vi "Gen VIs.vi"(8 "error in (no error)":errorcluster, 11 "Progress":refnum<vi>) -> (0 "error out":errorcluster, 3 "Progress (out)":refnum<vi>)   [LabVIEW 2020, in "WebServiceImporter.lvlib" / "VI Generator.lvlib"]
uses:
  <vilib>/Platform/WebService/VI Generator/VI Generator.lvlib
  <vilib>/Platform/WebService/Global/Const Strings.vi
  <vilib>/Platform/WebService/Main Panel/Pages/Progress/Progress.lvlib
  <vilib>/Platform/WebService/WebServiceImporter.lvlib
  <vilib>/Platform/WebService/ProxyDll Generator/ProxyDll Generator.lvlib
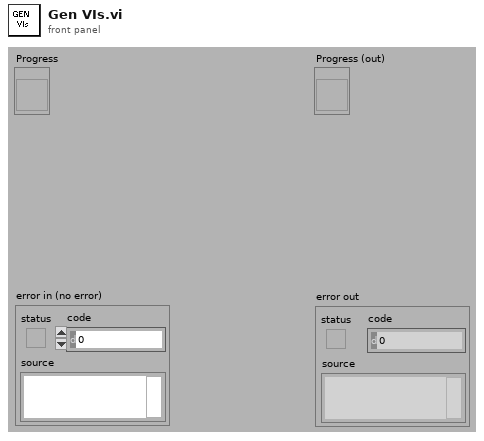
[diagram p1: front panel]
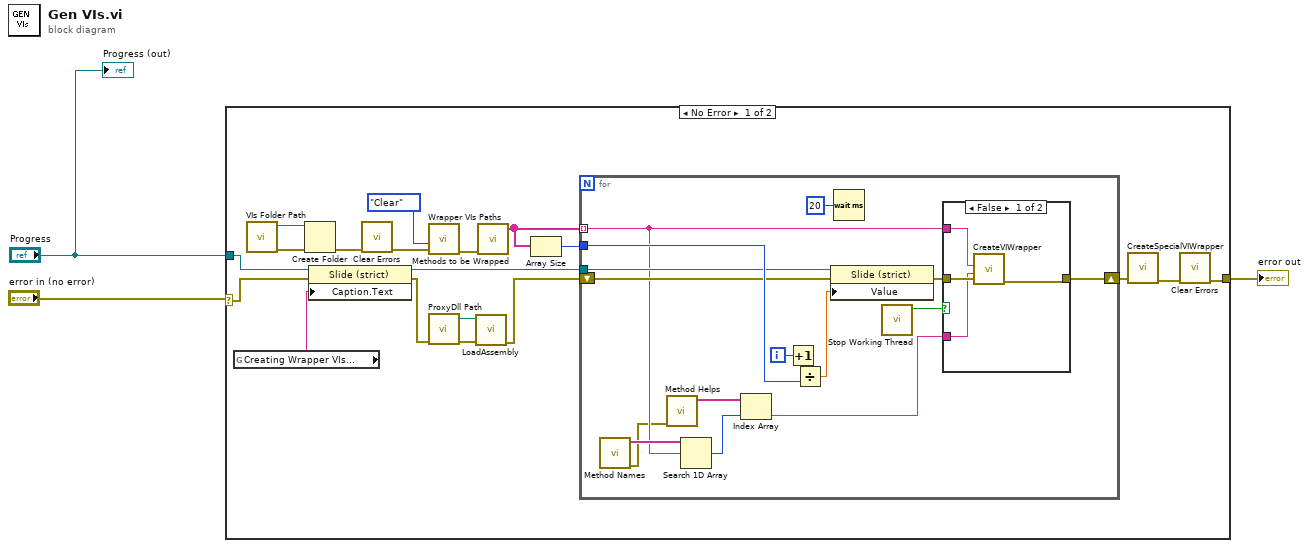
[diagram p0: block diagram]
diagram:
  n1 = case shown="No Error" "error in (no error)" {
    selector: "error in (no error)" -> [w18 w44]
    tunnel: "Progress" -> [w19 _]
    tunnel: [w13 w44] -> w2
    frame No Error {
      n2 = global read "Const Strings.vi" "Creating Wrapper VIs..."() -> (w10:string)
      n3 = call <vilib>:"VIs Folder Path.vi"() -> ("error out"=w7:errorcluster, "Path 2"=w6:path)  [unwired: 10 in]
      n4 = Create Folder(path (use dialog)=w6, error in=w7) -> (error out=w5:errorcluster)  [unwired: 1 in, 2 out]
      n5 = property class="Slide (strict)"(reference=w19, error in=w18, "Caption.Text"=w10) -> (reference out=w22:refnum<vi>, error out=w16:errorcluster)
      n6 = call <vilib>:"Clear Errors.vi"("error in (no error)"=w5) -> ("error out"=w4:errorcluster)  [unwired: 5 in, 1 out]
      n7 = call <vilib>:"Wrapper VIs Paths.vi"("error in (no error)"=w4, "Op"=enum16{"Get", "Add", "Clear"}."Clear") -> ("error out"=w11:errorcluster)  [unwired: 8 in, 1 out]
      n8 = call <vilib>:"ProxyDll Path.vi"("error in (no error)"=w16) -> ("error out"=w15:errorcluster, "ProxyDll Path (out)"=w17:path)  [unwired: 9 in]
      n9 = call <vilib>:"LoadAssembly.vi"("error in (no error)"=w15, "Assembly Path"=w17) -> ("error out"=w14:errorcluster)  [unwired: 9 in]
      n10 = call <vilib>:"Methods to be Wrapped.vi"("error in (no error)"=w11) -> ("Methods to be Wrapped (out)"=w21:string[])  [unwired: 9 in, 1 out]
      n11 = Array Size(array=w21) -> (size(s)=w20:i32)
      n12 = for {
        tunnel: w22 -> [w37]
        tunnel: w21 -> [w27] mode=indexing
        tunnel: w20 -> [w38]
        shift-right: [w33] -> w9
        shift-left: w14 -> [w35]
        i -> [w32]
        n13 = call <vilib>:"Method Names.vi"() -> ("error out"=w24:errorcluster, "Method Names (out)"=w28:string[])  [unwired: 10 in]
        n14 = call <vilib>:"Method Helps.vi"("error in (no error)"=w24) -> ("Method Helps (out)"=w26:string[])  [unwired: 9 in, 1 out]
        n15 = Search 1D Array(1D array=w28, element=w27) -> (index of element=w25:i32)  [unwired: 1 in]
        n16 = Index Array(array=w26, index=w25) -> (element=w23:string)
        n17 = Increment(x=w32) -> (x+1=w31:i32)
        n18 = Divide(x=w31, y=w38) -> (x/y=w36:dbl)
        n19 = property class="Slide (strict)"(reference=w37, error in=w35, "Value"=w36) -> (error out=w34:errorcluster)  [unwired: 1 out]
        n20 = Wait (ms)(milliseconds to wait=u32 20) -> ()  [unwired: 1 out]
        n21 = call <vilib>:"Stop Working Thread.vi"() -> ("Stop the working thread(out)"=w29:bool)  [unwired: 10 in, 1 out]
        n22 = case shown="False" w29 {
          tunnel: w27 -> [w41 _]
          tunnel: w34 -> [w42 w43]
          tunnel: [w40 w43] -> w33
          tunnel: w23 -> [w39 _]
          frame False {
            n23 = call <vilib>:"CreateVIWrapper.vi"("error in (no error)"=w42, "Method Help"=w39, "Method Name"=w41) -> ("error out"=w40:errorcluster)  [unwired: 7 in, 1 out]
          }
          frame True {
          }
        }
      }
      n24 = call <vilib>:"CreateSpecialVIWrapper.vi"("error in (no error)"=w9) -> ("error out"=w8:errorcluster)  [unwired: 10 in]
      n25 = call <vilib>:"Clear Errors.vi"("error in (no error)"=w8) -> ("error out"=w13:errorcluster)  [unwired: 5 in, 1 out]
    }
    frame Error {
    }
  }
  "error out" <- w2
  "Progress (out)" <- "Progress"
